vi "Field Draw Robots.vi"(3 "Draw Targets?":T1, 4 "our_robots":T2[](array[typedef]), 5 "Draw Number":bool=TRUE, 6 "color(black)":u32, 7 "IA Judge.Time":enum16{"Azul", "Amarelo"}(ring), 8 "Picture In":picture, 9 "Offset":cluster{"Width":dbl, "Height":dbl}, 10 "Scale":dbl, 11 "Detection Robots":T5[](array[typedef]) {"height" format="%+4.3f"; "pixel_y" format="%+4.3f"; "pixel_x" format="%+4.3f"; "orientation" format="%+4.3f"; "y" format="%+4.3f"; "confidence" format="%4.3f"; "x" format="%+4.3f"}) -> (0 "Picture Out":picture, 1 "Offset Out":cluster{"Width":dbl, "Height":dbl}, 2 "Scale Out":dbl)   [LabVIEW 2016]
uses:
  SSL Detection Robot.ctl
  <vilib>/Analysis/Matrix/Datatypes/RealMatrix.ctl
  Core/AI Robot.ctl
  Intel/Functions Enum.ctl
  Intel/AttackerStates.ctl
  DrawTargets.ctl
  <vilib>/Analysis/Matrix/NI_Matrix.lvlib
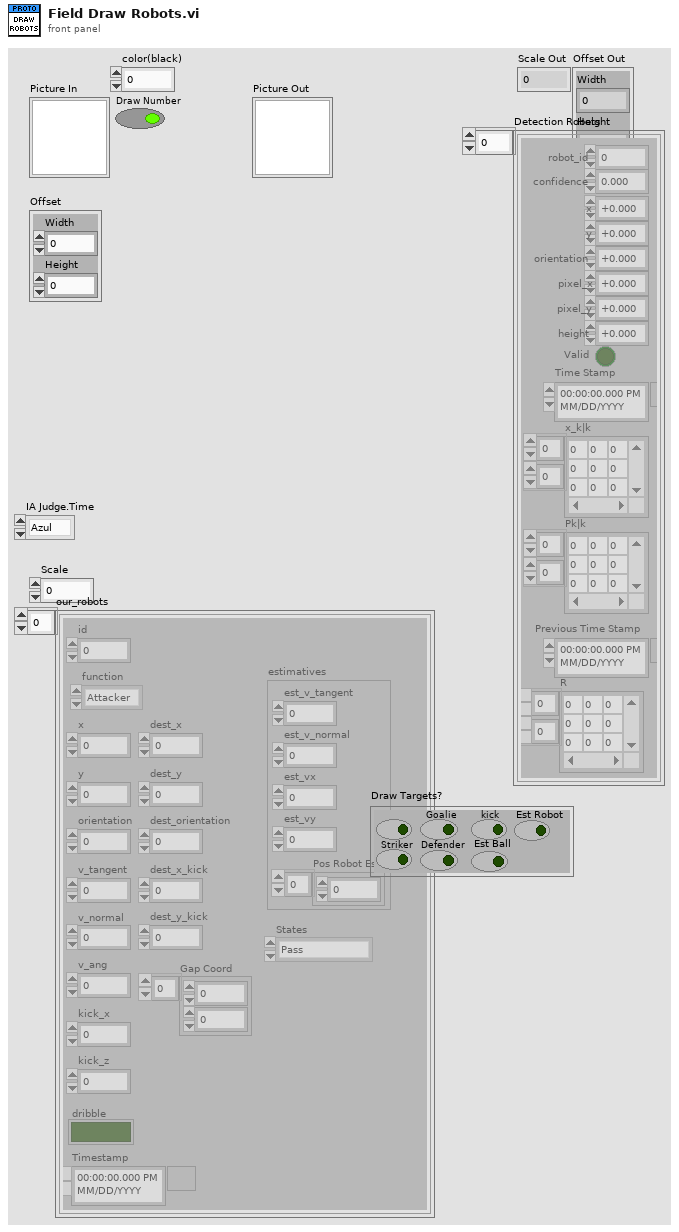
[diagram p1: front panel]
types:
  T1 = typedef "DrawTargets.ctl" = cluster{"Attacker":bool, "Striker":bool, "Goalie":bool, "Defender":bool, "kick":bool, "Est Ball":bool, "Est Robot":bool}
  T2 = typedef "AI Robot.ctl" = cluster{"id":u32, "function":T3, "x":dbl, "y":dbl, "orientation":dbl, "v_tangent":dbl, "v_normal":dbl, "v_ang":dbl, "kick_x":dbl, "kick_z":dbl, "dribble":bool, "Timestamp":timestamp, "dest_x":dbl, "dest_y":dbl, "dest_orientation":dbl, "estimatives":cluster{"est_v_tangent":dbl, "est_v_normal":dbl, "est_vx":dbl, "est_vy":dbl, "Pos Robot Est":dbl[]}, "dest_x_kick":dbl, "dest_y_kick":dbl, "Gap Coord":dbl[], "States":T4}
  T3 = typedef "Functions Enum.ctl" = enum16{"Attacker", "Goalie", "Defender", "Striker", "Goto 0", "Dummy", "Kicker", "ZigZag"}
  T4 = typedef "AttackerStates.ctl" = enum16{"Pass", "GoToTangent", "BallGetting", "GoToKick", ""}
  T5 = typedef "SSL Detection Robot.ctl" = cluster{"x":sgl, "robot_id":u32, "confidence":sgl, "y":sgl, "orientation":sgl, "pixel_x":sgl, "pixel_y":sgl, "height":sgl, "Valid":bool, "Time Stamp":timestamp, "x_k|k":T6, "Pk|k":T6, "Previous Time Stamp":timestamp, "R":T6}
  T6 = typedef "NI_Matrix.lvlib/RealMatrix.ctl" = dbl[][]
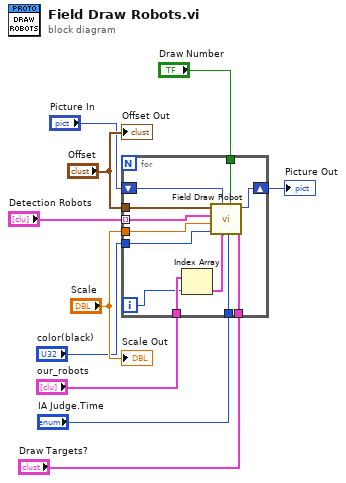
[diagram p0: block diagram]
diagram:
  n1 = for {
    tunnel: "Scale" -> [w22]
    tunnel: "Offset" -> [w20]
    shift-right: [w21] -> w5
    shift-left: "Picture In" -> [w19]
    tunnel: "color(black)" -> [w18]
    tunnel: "Detection Robots" -> [w17] mode=indexing
    tunnel: "Draw Number" -> [w16]
    tunnel: "our_robots" -> [w15]
    tunnel: "IA Judge.Time" -> [w12]
    tunnel: "Draw Targets?" -> [w11]
    i -> [w14]
    n2 = Index Array(array=w15, index=w14) -> (element=w13:T2)
    n3 = call "Field Draw Robot.vi"("Draw Targets?"=w11, "IA Judge.Time"=w12, "Draw Number"=w16, "Robot"=w13, "picture in"=w19, "color(black)"=w18, "Scale mm/pixel"=w22, "Detection Robot"=w17, "Offset"=w20) -> ("picture out"=w21:picture)  [unwired: 2 in]
  }
  "Picture Out" <- w5
  "Scale Out" <- "Scale"
  "Offset Out" <- "Offset"
